vi "Intan_binary_to_uV_offset_and_scale.vi"(3 "offset spacing factor":dbl=1.0, 4 "Yscale (uv/div)":dbl, 5 "ScaledData [Nchans x Nsamps]":dbl[][](array[numeric])) -> (0 "Nchannels":i32, 2 "Data4Display":dbl[][](array[numeric]))   [LabVIEW 2017]
doc: "Add baseline offsets to one scan of data points (1 samp x N chans) for clarity in visual display. Chan 1 has max offset (displayed on top), chan 32 on bottom with max negative offset.\n\nData is scaled according to uV/div value. \n\nOffsets are by default spacing of 1, but can be made closer or farther apart with 'offset factor'"
panel:
  out "iter":i32
  out "Sz init array":i32[](array[numeric])
  out "Nsamps":i32
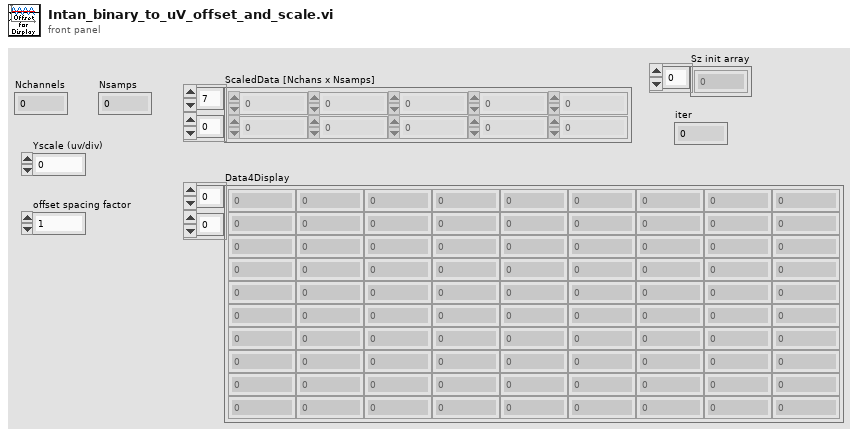
[diagram p1: front panel]
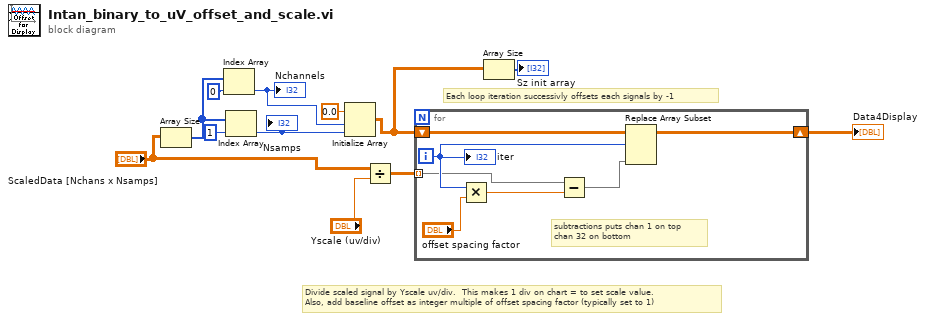
[diagram p0: block diagram]
diagram:
  # "Each loop iteration successivly offsets each signals by -1"
  # "Divide scaled signal by Yscale uv/div.  This makes 1 div on chart = to set scale value.\nAlso, add baseline offset as integer multiple of offset spacing factor (typically set to 1)"
  n1 = Array Size(array="ScaledData [Nchans x Nsamps]") -> (size(s)=w7:i32[])
  n2 = Index Array(array=w7, index=0) -> (element=w6:i32)
  "Nchannels" <- w6
  n3 = Index Array(array=w7, index=1) -> (element=w5:i32)
  "Nsamps" <- w5
  n4 = Initialize Array(0.0 ("element"), w6, w5) -> (w2:dbl[][])
  n5 = Divide(x="ScaledData [Nchans x Nsamps]", y="Yscale (uv/div)") -> (x/y=w10:dbl[][])
  n6 = for {
    shift-right: [w13] -> w4
    shift-left: w2 -> [w19]
    tunnel: w10 -> [w14] mode=indexing
    i -> [w15]
    # "subtractions puts chan 1 on top\nchan 32 on bottom"
    n7 = Multiply(x=w15, y="offset spacing factor") -> (x*y=w18:dbl)
    n8 = Subtract(x=w14, y=w18) -> (x-y=w17:dbl[])
    n9 = Replace Array Subset(array=w19, new element=w17, index (row)=w15) -> (w13:dbl[][])  [unwired: 1 in]
    "iter" <- w15
  }
  "Data4Display" <- w4
  n10 = Array Size(array=w2) -> (size(s)=→"Sz init array":i32[])
